vi "isEmpty.vi"(8 "error in (no error)":errorcluster, 11 "xwpfDocument.Element in":refnum<class "xwpfDocument.Element.lvclass">) -> (0 "error out":errorcluster, 2 "IsEmpty":bool, 3 "xwpfDocument.Element out":refnum<class "xwpfDocument.Element.lvclass">)   [LabVIEW 2017, in "Word_Specific.lvlib" / "xwpfDocument.Element.lvclass"]
uses:
  xwpfDocument.Element.lvclass
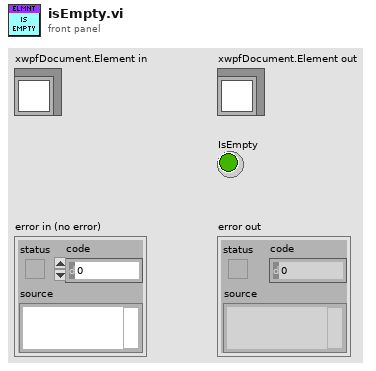
[diagram p1: front panel]
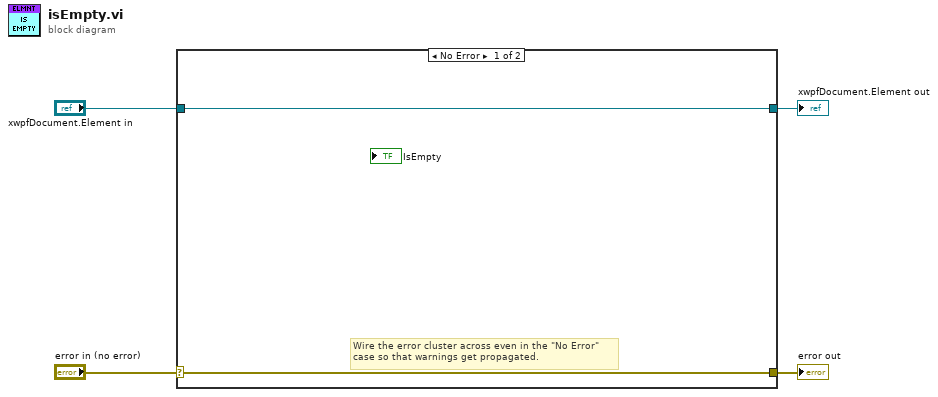
[diagram p0: block diagram]
diagram:
  n1 = case shown="No Error" "error in (no error)" {
    selector: "error in (no error)" -> [w5 w8]
    tunnel: [w5 w8] -> w3
    tunnel: [w6 w7] -> w1
    tunnel: "xwpfDocument.Element in" -> [w6 w7]
    frame No Error {
      # "Wire the error cluster across even in the \"No Error\"\ncase so that warnings get propagated."
    }
    frame Error {
    }
  }
  "error out" <- w3
  "xwpfDocument.Element out" <- w1
